vi "Delete Termination.vi"(0 "State in":refnum<class "State.lvclass">, 7 "termIndex":i32, 11 "error in (no error)":errorcluster) -> (4 "State out":refnum<class "State.lvclass">, 15 "error out":errorcluster)   [LabVIEW 2015, in "State.lvclass"]
uses:
  State.lvclass
  State.lvclass/State.ctl
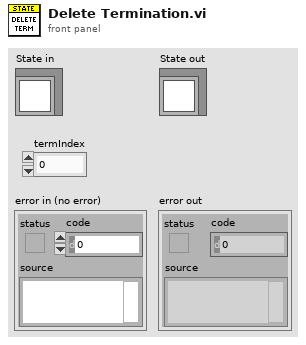
[diagram p1: front panel]
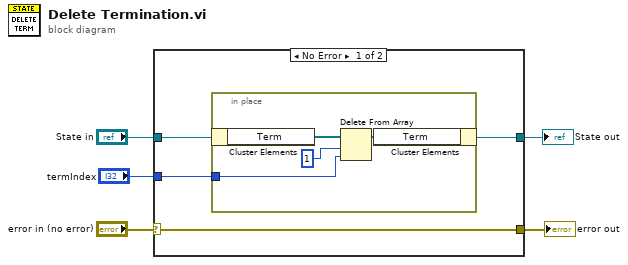
[diagram p0: block diagram]
diagram:
  n1 = case shown="No Error" "error in (no error)" {
    selector: "error in (no error)" -> [w9 w15]
    tunnel: [w9 w15] -> w4
    tunnel: "State in" -> [w8 w14]
    tunnel: "termIndex" -> [w7 _]
    tunnel: [w6 w14] -> w1
    frame No Error {
      n2 = in-place {
        in-place-border: w7 -> [w11]
        n3 = in-place-cluster #1(w8) -> ("Term"=w13:refnum<class "Termination.lvclass">[])
        n4 = Delete From Array(array=w13, length=1, index=w11) -> (array with subset deleted=w10:refnum<class "Termination.lvclass">[])  [unwired: 1 out]
        n5 = in-place-cluster #1("Term"=w10) -> (w6:refnum<class "State.lvclass">)
      }
    }
    frame Error {
    }
  }
  "error out" <- w4
  "State out" <- w1
